vi "Create.vi"(5 "Debug Flags":refnum<class "Debug Flags.lvclass">, 6 "framework id":i32, 7 "Plugin Configuration":T1={"name"="", "class"="", "cycle timing"={"priority"=0, "decimation"=1, "offset"=0}, "Transfer Groups"=[], "thread count"=0, "buffer converter settings"=[], "transceiver settings"=[]} {"Transfer Groups"."Transfers"."channels"."dst buffer offset" format="%d bytes"; "Transfer Groups"."Transfers"."channels"."src buffer offset" format="%d bytes"}, 8 "error in (no error)":errorcluster, 10 "component classes":refnum<class>[](array[class]), 11 "Transfer Groups":refnum<class "Transfer Group.lvclass">[](array[class])) -> (0 "error out":errorcluster, 3 "Plugin out":refnum<class "Plugin.lvclass">)   [LabVIEW 2017, in "DSF Core.lvlib" / "Plugin.lvclass"]
uses:
  Plugin.lvclass
  Transfer Group/Transfer Group.lvclass
  Timing/Timing.lvclass
  Thread/Plugin/Plugin Thread.lvclass
  Debug/Debug Flags/Debug Flags.lvclass
  Thread Pool/ID Pool.lvclass
  C:/Git/DSF/Data Sharing Framework/Source/Core/Engine/Classes/Thread Pool/Pool.lvclass
  DSF Configuration API/Public/Controls/DSF Timing Info.ctl
  DSF Core.lvlib
  DSF Configuration API/Public/Controls/DSF Direction.ctl
  DSF Configuration API/Public/Controls/DSF Byte Order.ctl
  DSF Configuration API/Public/Controls/DSF Data Type.ctl
  DSF Configuration API/Public/Controls/DSF Settings Info.ctl
  DSF Configuration API/Public/Controls/DSF Engine Channel Configuration.ctl
  DSF Configuration API/Public/Controls/DSF Engine Transfer Configuration.ctl
  DSF Configuration API/Public/Controls/DSF Engine Transfer Group Configuration.ctl
  DSF Configuration API/Public/Controls/DSF Engine Plugin Configuration.ctl
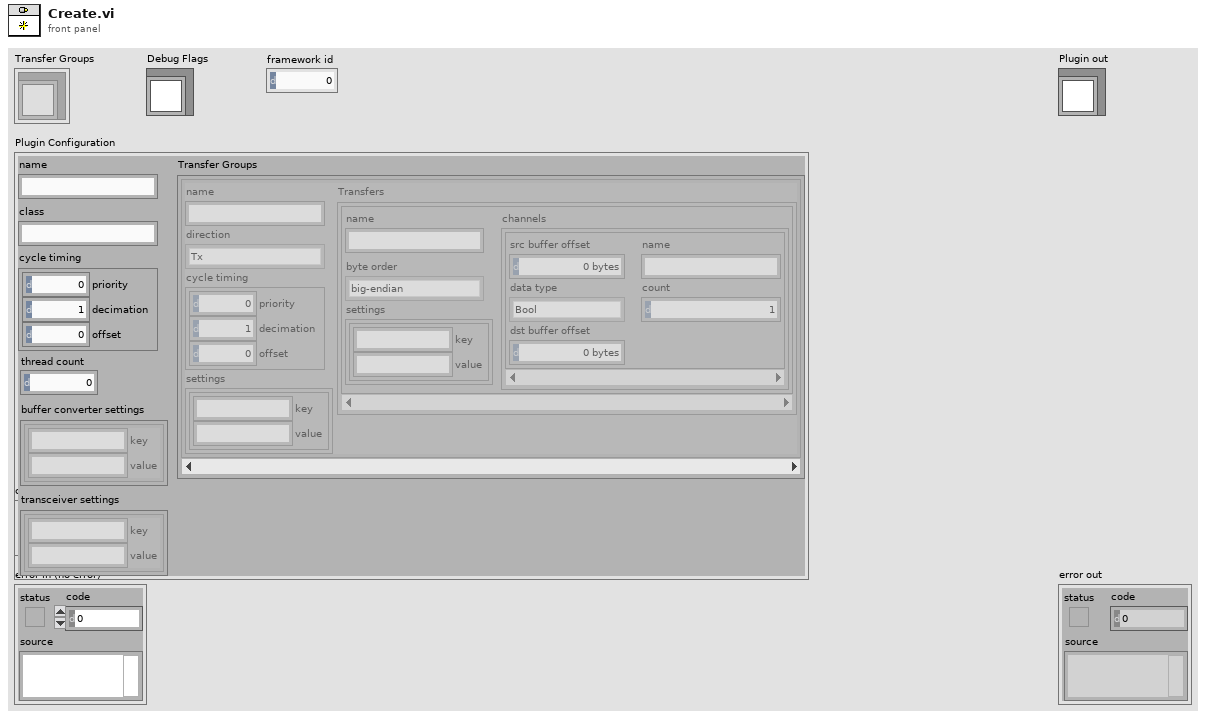
[diagram p1: front panel]
types:
  T1 = typedef "DSF Core.lvlib/DSF Engine Plugin Configuration.ctl" = cluster{"name":string, "class":string, "cycle timing":T2, "Transfer Groups":T3[], "thread count":i32, "buffer converter settings":T9, "transceiver settings":T9}
  T2 = typedef "DSF Core.lvlib/DSF Timing Info.ctl" = cluster{"priority":u64, "decimation":u64, "offset":u64}
  T3 = typedef "DSF Core.lvlib/DSF Engine Transfer Group Configuration.ctl" = cluster{"name":string, "direction":T4, "cycle timing":T2, "Transfers":T5[], "settings":T9}
  T4 = typedef "DSF Core.lvlib/DSF Direction.ctl" = enum8{"Tx", "Rx"}
  T5 = typedef "DSF Core.lvlib/DSF Engine Transfer Configuration.ctl" = cluster{"name":string, "byte order":T6, "channels":T7[], "settings":T9}
  T6 = typedef "DSF Core.lvlib/DSF Byte Order.ctl" = enum8{"big-endian", "little-endian"}
  T7 = typedef "DSF Core.lvlib/DSF Engine Channel Configuration.ctl" = cluster{"src buffer offset":u64, "name":string, "data type":T8, "count":u64, "dst buffer offset":u64}
  T8 = typedef "DSF Core.lvlib/DSF Data Type.ctl" = enum8{"Bool", "SGL", "DBL", "I8", "I16", "I32", "I64", "U8", "U16", "U32", "U64"}
  T9 = typedef "DSF Core.lvlib/DSF Settings Info.ctl" = cluster{"key":string, "value":string}[]
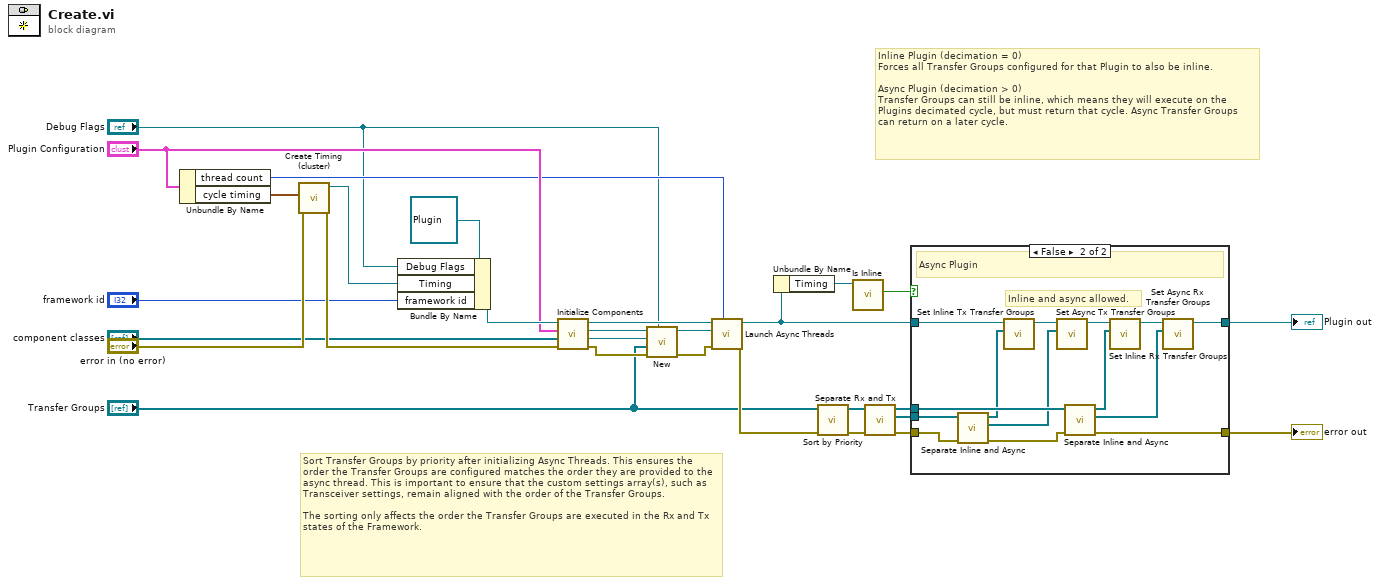
[diagram p0: block diagram]
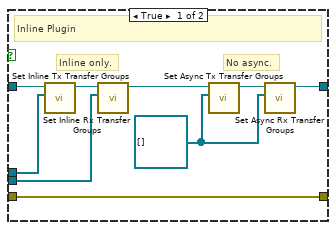
[diagram p2: hidden frame]
diagram:
  # "Sort Transfer Groups by priority after initializing Async Threads. This ensures the order the Transfer Groups are configured matches the order they are provided to the async thread. This is important to ensure that the custom settings array(s), such as Transceiver settings, remain aligned with the order of the Transfer Groups.\n\nThe sorting only affects the order the Transfer Groups are executed in the Rx and Tx states of the Framework."
  # "Inline Plugin (decimation = 0)\nForces all Transfer Groups configured for that Plugin to also be inline.\n\nAsync Plugin (decimation > 0)\nTransfer Groups can still be inline, which means they will execute on the Plugins decimated cycle, but must return that cycle. Async Transfer Groups can return on a later cycle."
  n1 = Unbundle By Name("Plugin Configuration") -> ("thread count"=w4:i32, "cycle timing"=w1:T2)
  n2 = call "Create Timing (cluster).vi"("error in (no error)"="error in (no error)", "cycle timing"=w1) -> ("error out"=w13:errorcluster, "Timing"=w18:refnum<class "Timing.lvclass">)  [unwired: 8 in]
  n3 = Bundle By Name(cluster=refnum<class "Plugin.lvclass"> refnum ("Plugin in"), "Debug Flags"="Debug Flags", "Timing"=w18, "framework id"="framework id") -> (w15:refnum<class "Plugin.lvclass">)
  n4 = call "Initialize Components.vi"("error in (no error)"=w13, "component classes"="component classes", "Plugin Configuration"="Plugin Configuration", "Plugin in"=w15) -> ("error out"=w8:errorcluster, "Buffer Converter"=w9:refnum<class "Buffer Converter.lvclass">, "Transceiver"=w10:refnum<class "Transceiver.lvclass">, "Plugin out"=w14:refnum<class "Plugin.lvclass">)  [unwired: 4 in]
  n5 = call "New.vi"("Thread ID Pool"="Debug Flags", "error in (no error)"=w8, "Transfer Groups"="Transfer Groups", "Buffer Converter"=w9, "Transceiver"=w10) -> ("error out"=w5:errorcluster, "Plugin Thread out"=w6:refnum<class "Plugin Thread.lvclass">)  [unwired: 4 in, 1 out]
  n6 = call "Launch Async Threads.vi"("thread count"=w4, "error in (no error)"=w5, "Plugin Thread"=w6, "Plugin in"=w14) -> ("error out"=w23:errorcluster, "Plugin out"=w17:refnum<class "Plugin.lvclass">)  [unwired: 6 in]
  n7 = Unbundle By Name(w17) -> ("Timing"=w16:refnum<class "Timing.lvclass">)
  n8 = call "Sort by Priority.vi"("error in (no error)"=w23, "Transfer Groups"="Transfer Groups") -> ("error out"=w29:errorcluster, "sorted Transfer Groups"=w28:refnum<class "Transfer Group.lvclass">[])  [unwired: 8 in]
  n9 = call "Is Inline.vi"("Timing in"=w16) -> ("inline?"=w21:bool)  [unwired: 9 in, 1 out]
  n10 = call "Separate Rx and Tx.vi"("error in (no error)"=w29, "Transfer Groups"=w28) -> ("error out"=w27:errorcluster, "Tx Transfer Groups"=w26:refnum<class "Transfer Group.lvclass">[], "Rx Transfer Groups"=w25:refnum<class "Transfer Group.lvclass">[])  [unwired: 7 in]
  n11 = case shown="False" w21 {
    tunnel: w27 -> [w36 w52]
    tunnel: w26 -> [w38 w51]
    tunnel: w25 -> [w37 w50]
    tunnel: w17 -> [w34 w45]
    tunnel: [w35 w44] -> w24
    tunnel: [w36 w43] -> w22
    frame True {
      w30 = refnum<class "Transfer Group.lvclass">[] [] ("Async Tx Transfer Groups")
      # "No async."
      # "Inline only."
      # "Inline Plugin"
      n12 = call "Set Inline Rx Transfer Groups.vi"("Inline Rx Transfer Groups"=w37, "Plugin in"=w34) -> ("Plugin out"=w33:refnum<class "Plugin.lvclass">)  [unwired: 9 in]
      n13 = call "Set Inline Tx Transfer Groups.vi"("Inline Tx Transfer Groups"=w38, "Plugin in"=w33) -> ("Plugin out"=w32:refnum<class "Plugin.lvclass">)  [unwired: 9 in]
      n14 = call "Set Async Tx Transfer Groups.vi"("Async Tx Transfer Groups"=w30, "Plugin in"=w32) -> ("Plugin out"=w31:refnum<class "Plugin.lvclass">)  [unwired: 9 in]
      n15 = call "Set Async Rx Transfer Groups.vi"("Async Rx Transfer Groups"=w30, "Plugin in"=w31) -> ("Plugin out"=w35:refnum<class "Plugin.lvclass">)  [unwired: 9 in]
    }
    frame False {
      # "Inline and async allowed."
      # "Async Plugin"
      n16 = call "Separate Inline and Async.vi"("error in (no error)"=w52, "Transfer Groups"=w51) -> ("error out"=w49:errorcluster, "Async Transfer Groups"=w41:refnum<class "Transfer Group.lvclass">[], "Inline Transfer Groups"=w42:refnum<class "Transfer Group.lvclass">[])  [unwired: 7 in]
      n17 = call "Set Inline Tx Transfer Groups.vi"("Inline Tx Transfer Groups"=w42, "Plugin in"=w45) -> ("Plugin out"=w48:refnum<class "Plugin.lvclass">)  [unwired: 9 in]
      n18 = call "Set Async Tx Transfer Groups.vi"("Async Tx Transfer Groups"=w41, "Plugin in"=w48) -> ("Plugin out"=w47:refnum<class "Plugin.lvclass">)  [unwired: 9 in]
      n19 = call "Separate Inline and Async.vi"("error in (no error)"=w49, "Transfer Groups"=w50) -> ("error out"=w43:errorcluster, "Async Transfer Groups"=w39:refnum<class "Transfer Group.lvclass">[], "Inline Transfer Groups"=w40:refnum<class "Transfer Group.lvclass">[])  [unwired: 7 in]
      n20 = call "Set Inline Rx Transfer Groups.vi"("Inline Rx Transfer Groups"=w40, "Plugin in"=w47) -> ("Plugin out"=w46:refnum<class "Plugin.lvclass">)  [unwired: 9 in]
      n21 = call "Set Async Rx Transfer Groups.vi"("Async Rx Transfer Groups"=w39, "Plugin in"=w46) -> ("Plugin out"=w44:refnum<class "Plugin.lvclass">)  [unwired: 9 in]
    }
  }
  "error out" <- w22
  "Plugin out" <- w24
